vi "FTW-Test-Reflection-Datatypes.vi"() -> (0 "Test Result":errorcluster)   [LabVIEW 2014]
uses:
  src/core/reflection/FTW-Reflection-Types.ctl
  sandbox/deprecated/FTW-Collection-KeyValuePair.ctl
  src/core/actor/message/FTW-Message.lvclass
  src/core/database/FTW-SQLite-AccessMode.ctl
  src/core/error/FTW-ERR-ThrowError.vi
  src/core/error/FTW-ERR-Assert-DeveloperError.vi
  src/core/error/FTW-ERR-CallChain.vi
  src/core/string/FTW-STR-ReplaceWhitespace.vi
  src/core/database/FTW-SQLite-Connector.lvclass
panel:
  in  "DynamicData":dynamicdata(waveform)
  out "Results Array":T2(array[cluster])
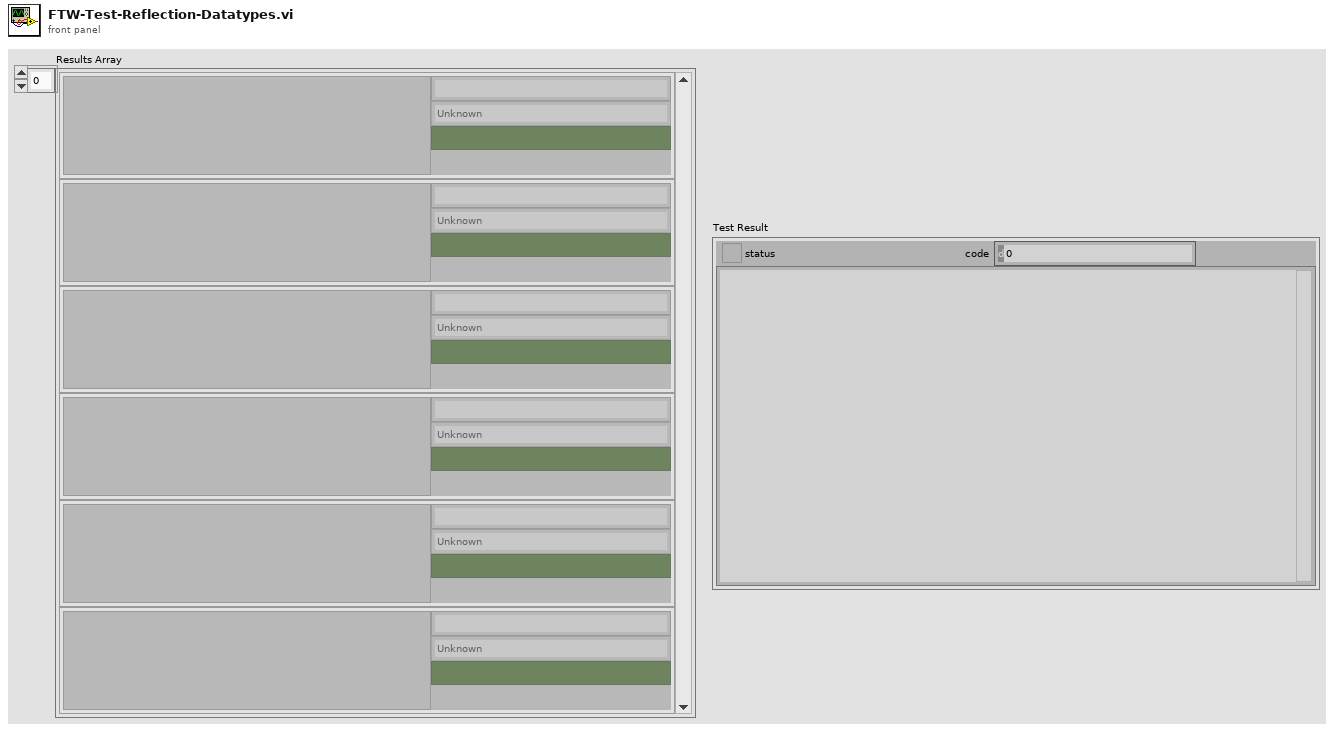
[diagram p1: front panel]
types:
  T1 = typedef "FTW-Reflection-Types.ctl" = enum16{"Unknown", "Void", "Array", "Cluster", "LVObject", "Boolean", "I8", "I16", "I32", "I64", "U8", "U16", "U32", "U64", "SGL", "DBL", "EXT", "CSG", "CDB", "CXT", "FXP", "EnumU8", "EnumU16", "EnumU32", "EnumU64", "SGLwithUnit", "DBLwithUnit", "EXTwithUnit", "CSGwithUnit", "CDBwithUnit", "CXTwithUnit", "String", "Path", "Picture", "Tag", "LVVariant", "Timestamp", "WaveformI8", "WaveformI16", "WaveformI32", "WaveformI64", "WaveformU8", "WaveformU16", "WaveformU32", "WaveformU64", "WaveformSGL", "WaveformDBL", "WaveformEXT", "WaveformCSG", "WaveformCDB", "WaveformCXT", "WaveformDigital", "WaveformUnknownType", "DigitalData", "DynamicData", "ExternalData", "FileByteStream", "TDMStream", "dotNET", "ActiveX", "VIServerReference", "VIReference", "ApplicationInstance", "Menu", "ConnectionDataSocket", "ConnectionVISA", "ConnectionBluetooth", "ConnectionIrDA", "ConnectionTCP", "ConnectionUDP", "ConnectionHTTPClient", "ConnectionFTP", "Occurrence", "Notifier", "Queue", "Rendezvous", "Semaphore", "RTFIFO", "EventPublisher", "EventRegistration", "EventCallback", "DataValueReference", "GenericClass", "GenericClassTag", "GenericClassDeepCopy", "GenericClassFlattened", "GenericClassTagFlattened", "GenericReferenceType", "WindowsRegistry", "OverloadedDatalogRef", "ReferenceUnknownType"}
  T2 = cluster{"Variant":variant, "xml string":string, "LabVIEW Type":T1, "Pass?":bool}[]
  T3 = typedef "Rendezvous RefNum" = refnum<k1>
  T4 = typedef "Semaphore RefNum" = refnum<k1>
  T5 = typedef "FTW-SQLite-Connector.lvclass/FTW-SQLite-AccessMode.ctl" = enum16{"Read", "Read/Write", "Read/Write/Create"}
  T6 = typedef "FTW-Collection-KeyValuePair.ctl" = cluster{"Key":string, "Value":string}
  T7 = cluster{"Variant":variant, "Match":string, "LabVIEW Type":T1, "Status OK?":bool}
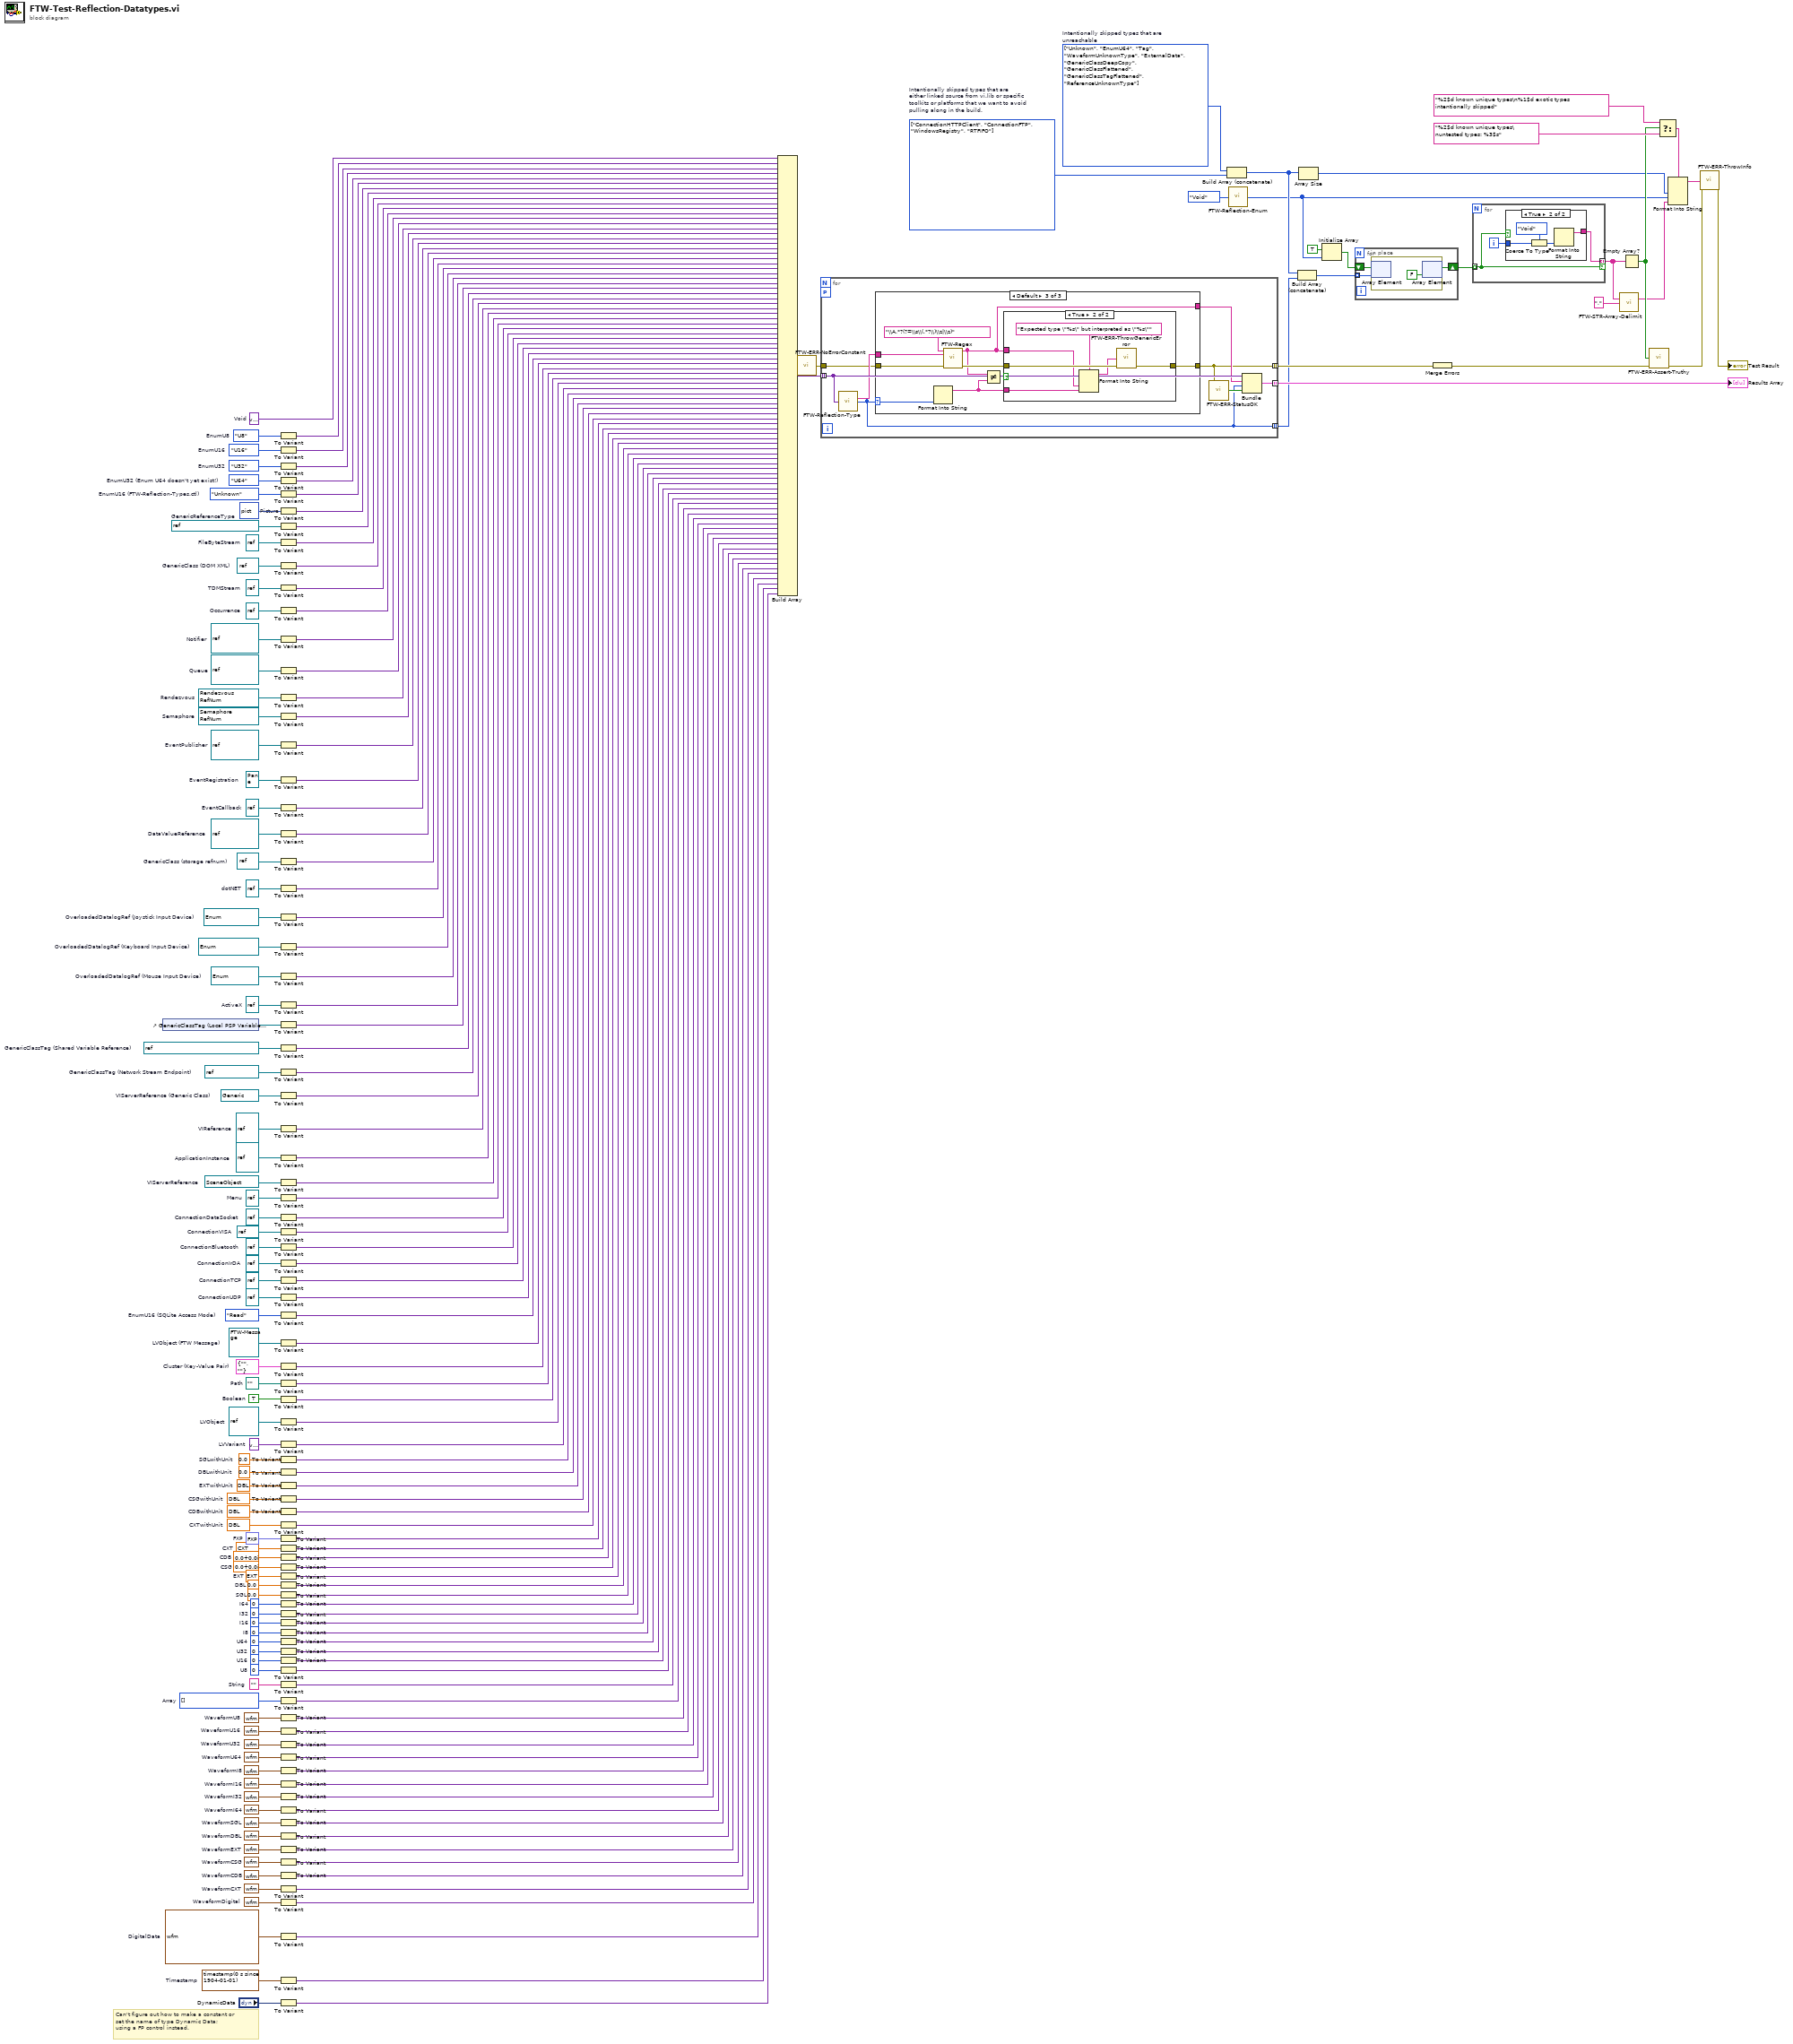
[diagram p0: block diagram]
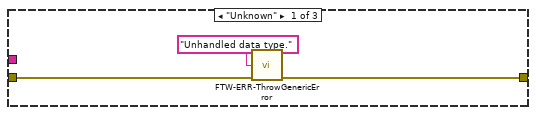
[diagram p3: hidden frame]
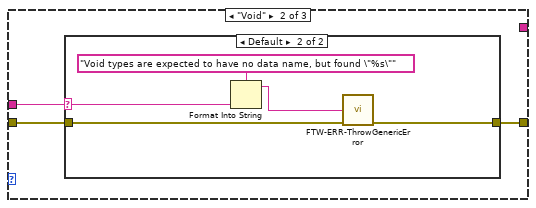
[diagram p4: hidden frame]
diagram:
  w19 = T1[] [enum."ConnectionHTTPClient", enum."ConnectionFTP", enum."WindowsRegistry", enum."RTFIFO"] items=["Unknown", "Void", "Array", "Cluster", "LVObject", "Boolean", "I8", "I16", "I32", "I64", "U8", "U16", "U32", "U64", "SGL", "DBL", "EXT", "CSG", "CDB", "CXT", "FXP", "EnumU8", "EnumU16", "EnumU32", "EnumU64", "SGLwithUnit", "DBLwithUnit", "EXTwithUnit", "CSGwithUnit", "CDBwithUnit", "CXTwithUnit", "String", "Path", "Picture", "Tag", "LVVariant", "Timestamp", "WaveformI8", "WaveformI16", "WaveformI32", "WaveformI64", "WaveformU8", "WaveformU16", "WaveformU32", "WaveformU64", "WaveformSGL", "WaveformDBL", "WaveformEXT", "WaveformCSG", "WaveformCDB", "WaveformCXT", "WaveformDigital", "WaveformUnknownType", "DigitalData", "DynamicData", "ExternalData", "FileByteStream", "TDMStream", "dotNET", "ActiveX", "VIServerReference", "VIReference", "ApplicationInstance", "Menu", "ConnectionDataSocket", "ConnectionVISA", "ConnectionBluetooth", "ConnectionIrDA", "ConnectionTCP", "ConnectionUDP", "ConnectionHTTPClient", "ConnectionFTP", "Occurrence", "Notifier", "Queue", "Rendezvous", "Semaphore", "RTFIFO", "EventPublisher", "EventRegistration", "EventCallback", "DataValueReference", "GenericClass", "GenericClassTag", "GenericClassDeepCopy", "GenericClassFlattened", "GenericClassTagFlattened", "GenericReferenceType", "WindowsRegistry", "OverloadedDatalogRef", "ReferenceUnknownType"]  # Intentionally skipped types that are either linked source from vi.lib or specific toolkits or platforms that we want to avoid pulling along in the build.
  w20 = T1[] [enum."Unknown", enum."EnumU64", enum."Tag", enum."WaveformUnknownType", enum."ExternalData", enum."GenericClassDeepCopy", enum."GenericClassFlattened", enum."GenericClassTagFlattened", enum."ReferenceUnknownType"] items=["Unknown", "Void", "Array", "Cluster", "LVObject", "Boolean", "I8", "I16", "I32", "I64", "U8", "U16", "U32", "U64", "SGL", "DBL", "EXT", "CSG", "CDB", "CXT", "FXP", "EnumU8", "EnumU16", "EnumU32", "EnumU64", "SGLwithUnit", "DBLwithUnit", "EXTwithUnit", "CSGwithUnit", "CDBwithUnit", "CXTwithUnit", "String", "Path", "Picture", "Tag", "LVVariant", "Timestamp", "WaveformI8", "WaveformI16", "WaveformI32", "WaveformI64", "WaveformU8", "WaveformU16", "WaveformU32", "WaveformU64", "WaveformSGL", "WaveformDBL", "WaveformEXT", "WaveformCSG", "WaveformCDB", "WaveformCXT", "WaveformDigital", "WaveformUnknownType", "DigitalData", "DynamicData", "ExternalData", "FileByteStream", "TDMStream", "dotNET", "ActiveX", "VIServerReference", "VIReference", "ApplicationInstance", "Menu", "ConnectionDataSocket", "ConnectionVISA", "ConnectionBluetooth", "ConnectionIrDA", "ConnectionTCP", "ConnectionUDP", "ConnectionHTTPClient", "ConnectionFTP", "Occurrence", "Notifier", "Queue", "Rendezvous", "Semaphore", "RTFIFO", "EventPublisher", "EventRegistration", "EventCallback", "DataValueReference", "GenericClass", "GenericClassTag", "GenericClassDeepCopy", "GenericClassFlattened", "GenericClassTagFlattened", "GenericReferenceType", "WindowsRegistry", "OverloadedDatalogRef", "ReferenceUnknownType"]  # Intentionally skipped types that are unreachable
  w24 = u8[] []  # Array
  w23 = ""  # String
  w12 = T3 refnum items=["rendezvous"]  # Rendezvous
  w11 = T4 refnum items=["semaphore"]  # Semaphore
  w27 = enum32{"U64"}."U64"  # EnumU32 (Enum U64 doesn't yet exist!)
  w37 = FTW-SQLite-AccessMode."Read"  # EnumU16 (SQLite Access Mode)
  w38 = refnum<class "FTW-Message.lvclass"> refnum  # LVObject (FTW Message)
  w41 = digitalwaveform {"t0"=timestamp(0 s since 1904-01-01), "dt"=0.0, "Y"={"transitions"=[], "data"=[]}}  # WaveformDigital
  w42 = waveform(cxt) {"t0"=timestamp(0 s since 1904-01-01), "dt"=1.0, "Y"=[]}  # WaveformCXT
  w43 = waveform(cdb) {"t0"=timestamp(0 s since 1904-01-01), "dt"=1.0, "Y"=[]}  # WaveformCDB
  w44 = waveform(csg) {"t0"=timestamp(0 s since 1904-01-01), "dt"=1.0, "Y"=[]}  # WaveformCSG
  w45 = waveform(ext) {"t0"=timestamp(0 s since 1904-01-01), "dt"=1.0, "Y"=[]}  # WaveformEXT
  w46 = waveform(dbl) {"t0"=timestamp(0 s since 1904-01-01), "dt"=1.0, "Y"=[]}  # WaveformDBL
  w47 = waveform(sgl) {"t0"=timestamp(0 s since 1904-01-01), "dt"=1.0, "Y"=[]}  # WaveformSGL
  w48 = waveform(i64) {"t0"=timestamp(0 s since 1904-01-01), "dt"=1.0, "Y"=[]}  # WaveformI64
  w49 = waveform(i32) {"t0"=timestamp(0 s since 1904-01-01), "dt"=1.0, "Y"=[]}  # WaveformI32
  w50 = waveform(i16) {"t0"=timestamp(0 s since 1904-01-01), "dt"=1.0, "Y"=[]}  # WaveformI16
  w54 = waveform(i8) {"t0"=timestamp(0 s since 1904-01-01), "dt"=1.0, "Y"=[]}  # WaveformI8
  w55 = waveform(u64) {"t0"=timestamp(0 s since 1904-01-01), "dt"=1.0, "Y"=[]}  # WaveformU64
  w53 = waveform(u32) {"t0"=timestamp(0 s since 1904-01-01), "dt"=1.0, "Y"=[]}  # WaveformU32
  w52 = waveform(u16) {"t0"=timestamp(0 s since 1904-01-01), "dt"=1.0, "Y"=[]}  # WaveformU16
  w51 = waveform(u8) {"t0"=timestamp(0 s since 1904-01-01), "dt"=1.0, "Y"=[]}  # WaveformU8
  w2 = variant  # Void
  w129 = refnum<k31> refnum  # ConnectionBluetooth
  w100 = enum32{"U32"}."U32"  # EnumU32
  w99 = enum16{"U16"}."U16"  # EnumU16
  w98 = enum8{"U8"}."U8"  # EnumU8
  w133 = TRUE  # Boolean
  w135 = path ""  # Path
  w101 = FTW-Reflection-Types."Unknown"  # EnumU16 (FTW-Reflection-Types.ctl)
  w109 = refnum<event-registration> refnum  # EventRegistration
  w134 = T6 {"Key"="", "Value"=""}  # Cluster (Key-Value Pair)
  w132 = refnum<k16> refnum  # ConnectionUDP
  w131 = refnum<k5> refnum  # ConnectionTCP
  w127 = refnum<k13> refnum  # ConnectionDataSocket
  w126 = refnum<k9> refnum  # Menu
  w111 = refnum<data-value> refnum  # DataValueReference
  w130 = refnum<k19> refnum  # ConnectionIrDA
  w102 = picture data[5B]  # Picture
  w125 = refnum<vi> refnum  # VIServerReference
  w123 = refnum<vi> refnum  # ApplicationInstance
  w124 = refnum<vi> refnum  # VIReference
  w122 = refnum<vi> refnum  # VIServerReference (Generic Class)
  w121 = refnum<k21> "localhost"  # GenericClassTag (Network Stream Endpoint)
  w112 = refnum<k27> refnum  # EventCallback
  w110 = refnum<user-event> refnum  # EventPublisher
  w107 = refnum<k4> refnum  # Occurrence
  w16 = refnum<queue> refnum  # Queue
  w108 = refnum<notifier> refnum  # Notifier
  w120 = refnum<k21> "ni.var.psp://localhost/System"  # GenericClassTag (Shared Variable Reference)
  w118 = refnum<k7> refnum  # ActiveX
  w117 = refnum<k1> refnum items=["MOUSE"]  # OverloadedDatalogRef (Mouse Input Device)
  w115 = refnum<k1> refnum items=["KEYBOARD"]  # OverloadedDatalogRef (Keyboard Input Device)
  w116 = refnum<k1> refnum items=["JOYSTICK"]  # OverloadedDatalogRef (Joystick Input Device)
  w113 = refnum<k24> refnum  # dotNET
  w114 = refnum<k20> refnum  # GenericClass (storage refnum)
  w106 = refnum<k34> refnum  # TDMStream
  w103 = refnum<k0> refnum  # GenericReferenceType
  w128 = refnum<visa-resource-name> refnum  # ConnectionVISA
  w105 = refnum<k20> refnum  # GenericClass (DOM XML)
  w104 = refnum<file> refnum  # FileByteStream
  w137 = refnum<class> refnum  # LVObject
  w139 = variant  # LVVariant
  w151 = cxt[unit] 0.0+0.0i  # CXTwithUnit
  w150 = cdb[unit] 0.0+0.0i  # CDBwithUnit
  w149 = csg[unit] 0.0+0.0i  # CSGwithUnit
  w148 = ext[unit] 0.0  # EXTwithUnit
  w147 = dbl[unit] 0.0  # DBLwithUnit
  w146 = sgl[unit] 0.0  # SGLwithUnit
  w198 = timestamp(0 s since 1904-01-01)  # Timestamp
  w168 = cxt 0.0+0.0i  # CXT
  w169 = cdb 0.0+0.0i  # CDB
  w170 = csg 0.0+0.0i  # CSG
  w167 = fxp<+/-,64,1024> 0.0  # FXP
  w171 = ext 0.0  # EXT
  w172 = 0.0  # DBL
  w173 = sgl 0.0  # SGL
  w174 = i64 0  # I64
  w175 = 0  # I32
  w176 = i16 0  # I16
  w177 = i8 0  # I8
  w178 = u64 0  # U64
  w179 = u32 0  # U32
  w180 = u16 0  # U16
  w181 = u8 0  # U8
  w201 = digitaldata {"transitions"=[], "data"=[]}  # DigitalData
  # "Can't figure out how to make a constant or\nset the name of type Dynamic Data;\nusing a FP control instead."
  n1 = control-ref of="GenericClassTag (Local PSP Variable Engine)"() -> (w119:refnum<k21>)
  n2 = To Variant(anything=w98) -> (Variant=w1:variant)
  n3 = To Variant(anything=w99) -> (Variant=w57:variant)
  n4 = To Variant(anything=w100) -> (Variant=w25:variant)
  n5 = To Variant(anything=w27) -> (Variant=w26:variant)
  n6 = To Variant(anything=w101) -> (Variant=w58:variant)
  n7 = To Variant(anything=w102) -> (Variant=w59:variant)
  n8 = To Variant(anything=w103) -> (Variant=w60:variant)
  n9 = To Variant(anything=w104) -> (Variant=w61:variant)
  n10 = To Variant(anything=w105) -> (Variant=w62:variant)
  n11 = To Variant(anything=w106) -> (Variant=w63:variant)
  n12 = To Variant(anything=w107) -> (Variant=w64:variant)
  n13 = To Variant(anything=w108) -> (Variant=w65:variant)
  n14 = To Variant(anything=w16) -> (Variant=w66:variant)
  n15 = To Variant(anything=w12) -> (Variant=w67:variant)
  n16 = To Variant(anything=w11) -> (Variant=w68:variant)
  n17 = To Variant(anything=w110) -> (Variant=w69:variant)
  n18 = To Variant(anything=w109) -> (Variant=w70:variant)
  n19 = To Variant(anything=w112) -> (Variant=w71:variant)
  n20 = To Variant(anything=w111) -> (Variant=w72:variant)
  n21 = To Variant(anything=w114) -> (Variant=w73:variant)
  n22 = To Variant(anything=w113) -> (Variant=w74:variant)
  n23 = To Variant(anything=w116) -> (Variant=w75:variant)
  n24 = To Variant(anything=w115) -> (Variant=w76:variant)
  n25 = To Variant(anything=w117) -> (Variant=w77:variant)
  n26 = To Variant(anything=w118) -> (Variant=w78:variant)
  n27 = To Variant(anything=w119) -> (Variant=w79:variant)
  n28 = To Variant(anything=w120) -> (Variant=w80:variant)
  n29 = To Variant(anything=w121) -> (Variant=w81:variant)
  n30 = To Variant(anything=w122) -> (Variant=w82:variant)
  n31 = To Variant(anything=w124) -> (Variant=w83:variant)
  n32 = To Variant(anything=w123) -> (Variant=w84:variant)
  n33 = To Variant(anything=w125) -> (Variant=w85:variant)
  n34 = To Variant(anything=w126) -> (Variant=w86:variant)
  n35 = To Variant(anything=w127) -> (Variant=w87:variant)
  n36 = To Variant(anything=w128) -> (Variant=w88:variant)
  n37 = To Variant(anything=w129) -> (Variant=w89:variant)
  n38 = To Variant(anything=w130) -> (Variant=w90:variant)
  n39 = To Variant(anything=w131) -> (Variant=w91:variant)
  n40 = To Variant(anything=w132) -> (Variant=w92:variant)
  n41 = To Variant(anything=w37) -> (Variant=w93:variant)
  n42 = To Variant(anything=w38) -> (Variant=w94:variant)
  n43 = To Variant(anything=w134) -> (Variant=w95:variant)
  n44 = To Variant(anything=w135) -> (Variant=w96:variant)
  n45 = To Variant(anything=w133) -> (Variant=w97:variant)
  n46 = To Variant(anything=w137) -> (Variant=w136:variant)
  n47 = To Variant(anything=w139) -> (Variant=w138:variant)
  n48 = To Variant(anything=w146) -> (Variant=w140:variant)
  n49 = To Variant(anything=w147) -> (Variant=w141:variant)
  n50 = To Variant(anything=w148) -> (Variant=w142:variant)
  n51 = To Variant(anything=w149) -> (Variant=w143:variant)
  n52 = To Variant(anything=w150) -> (Variant=w144:variant)
  n53 = To Variant(anything=w151) -> (Variant=w145:variant)
  n54 = To Variant(anything=w167) -> (Variant=w152:variant)
  n55 = To Variant(anything=w168) -> (Variant=w153:variant)
  n56 = To Variant(anything=w169) -> (Variant=w154:variant)
  n57 = To Variant(anything=w170) -> (Variant=w155:variant)
  n58 = To Variant(anything=w171) -> (Variant=w156:variant)
  n59 = To Variant(anything=w172) -> (Variant=w157:variant)
  n60 = To Variant(anything=w173) -> (Variant=w158:variant)
  n61 = To Variant(anything=w174) -> (Variant=w159:variant)
  n62 = To Variant(anything=w175) -> (Variant=w160:variant)
  n63 = To Variant(anything=w176) -> (Variant=w161:variant)
  n64 = To Variant(anything=w177) -> (Variant=w162:variant)
  n65 = To Variant(anything=w178) -> (Variant=w163:variant)
  n66 = To Variant(anything=w179) -> (Variant=w164:variant)
  n67 = To Variant(anything=w180) -> (Variant=w165:variant)
  n68 = To Variant(anything=w181) -> (Variant=w166:variant)
  n69 = To Variant(anything=w23) -> (Variant=w22:variant)
  n70 = To Variant(anything=w24) -> (Variant=w21:variant)
  n71 = To Variant(anything=w51) -> (Variant=w197:variant)
  n72 = To Variant(anything=w52) -> (Variant=w196:variant)
  n73 = To Variant(anything=w53) -> (Variant=w195:variant)
  n74 = To Variant(anything=w55) -> (Variant=w194:variant)
  n75 = To Variant(anything=w54) -> (Variant=w193:variant)
  n76 = To Variant(anything=w50) -> (Variant=w192:variant)
  n77 = To Variant(anything=w49) -> (Variant=w191:variant)
  n78 = To Variant(anything=w48) -> (Variant=w190:variant)
  n79 = To Variant(anything=w47) -> (Variant=w189:variant)
  n80 = To Variant(anything=w46) -> (Variant=w188:variant)
  n81 = To Variant(anything=w45) -> (Variant=w187:variant)
  n82 = To Variant(anything=w44) -> (Variant=w186:variant)
  n83 = To Variant(anything=w43) -> (Variant=w185:variant)
  n84 = To Variant(anything=w42) -> (Variant=w184:variant)
  n85 = To Variant(anything=w41) -> (Variant=w183:variant)
  n86 = To Variant(anything=w201) -> (Variant=w182:variant)
  n87 = To Variant(anything=w198) -> (Variant=w56:variant)
  n88 = To Variant(anything="DynamicData") -> (Variant=w40:variant)
  n89 = Build Array(w2, w1, w57, w25, w26, w58, w59, w60, w61, w62, w63, w64, w65, w66, w67, w68, w69, w70, w71, w72, w73, w74, w75, w76, w77, w78, w79, w80, w81, w82, w83, w84, w85, w86, w87, w88, w89, w90, w91, w92, w93, w94, w95, w96, w97, w136, w138, w140, w141, w142, w143, w144, w145, w152, w153, w154, w155, w156, w157, w158, w159, w160, w161, w162, w163, w164, w165, w166, w22, w21, w197, w196, w195, w194, w193, w192, w191, w190, w189, w188, w187, w186, w185, w184, w183, w182, w56, w40) -> (w199:variant[])
  n90 = call "FTW-ERR-NoErrorConstant.vi"() -> ("no error"=w36:errorcluster)
  n91 = for {
    tunnel: w199 -> [w208] mode=indexing
    tunnel: [w209] -> w200 mode=indexing
    tunnel: w36 -> [w206]
    workers-P: _ -> [_]
    tunnel: [w204] -> w35 mode=indexing
    tunnel: [w202] -> w10 mode=indexing
    n92 = call "FTW-Reflection-Type.vi"("Anything"=w208) -> ("Data Name"=w207:string, "LabVIEW Type"=w202:T1)  [unwired: 12 in, 1 out]
    n93 = case shown="Default" w202 {
      selector: w202 -> [_ _ w227]
      tunnel: w207 -> [_ w213 w230]
      tunnel: w206 -> [w211 w215 w229]
      tunnel: [w210 w214 w224] -> w204
      tunnel: [_ _ w222] -> w205
      frame "Unknown" {
        n94 = call "FTW-ERR-ThrowGenericError.vi"("Error Message"="Unhandled data type.", "error in"=w211) -> ("error out"=w210:errorcluster)  [unwired: 13 in]
      }
      frame "Void" {
        n95 = case shown="Default" w213 {
          selector: w213 -> [_ w217]
          tunnel: w215 -> [w216 w221]
          tunnel: [w216 w220] -> w214
          frame "" {
          }
          frame Default {
            n96 = Format Into String(format string="Void types are expected to have no data name, but found \"%s\"", w217) -> (resulting string=w218:string)  [unwired: 2 in, 1 out]
            n97 = call "FTW-ERR-ThrowGenericError.vi"("Error Message"=w218, "error in"=w221) -> ("error out"=w220:errorcluster)  [unwired: 13 in]
          }
        }
      }
      frame Default {
        n98 = Format Into String(w227) -> (resulting string=w223:string)  [unwired: 3 in, 1 out]
        n99 = call "FTW-Regex.vi"("Regular Expression"="\\A.*?(?=\\s\\(.*?\\)\\z|\\z)", "Input String"=w230, "error in"=w229) -> ("Match"=w222:string, "error out"=w225:errorcluster)  [unwired: 8 in, 3 out]
        n100 = Not Equal?(x=w222, y=w223) -> (x != y?=w226:bool)
        n101 = case shown="True" w226 {
          tunnel: w225 -> [w231 w237]
          tunnel: [w231 w236] -> w224
          tunnel: w222 -> [_ w235]
          tunnel: w223 -> [_ w234]
          frame False {
          }
          frame True {
            n102 = Format Into String(format string="Expected type \"%s\" but interpreted as \"%s\"", w235, w234) -> (resulting string=w232:string)  [unwired: 2 in, 1 out]
            n103 = call "FTW-ERR-ThrowGenericError.vi"("Error Message"=w232, "error in"=w237) -> ("error out"=w236:errorcluster)  [unwired: 13 in]
          }
        }
      }
    }
    n104 = call "FTW-ERR-StatusOK.vi"("error to check"=w204) -> ("Status OK?"=w203:bool)
    n105 = Bundle("Variant"=w208, "Match"=w205, "LabVIEW Type"=w202, "Status OK?"=w203) -> (w209:T7)  [unwired: 1 in]
  }
  "Results Array" <- w200
  n106 = Build Array (concatenate)(w20, w19) -> (w17:T1[])
  n107 = call "FTW-Reflection-Enum.vi"("Enum"=FTW-Reflection-Types."Void" ("y")) -> ("Number of Items"=w4:i32)  [unwired: 12 in, 2 out]
  n108 = Build Array (concatenate)(w17, w10) -> (w18:T1[])
  n109 = Array Size(array=w17) -> (size(s)=w3:i32)
  n110 = Initialize Array(TRUE, w4) -> (w29:bool[])
  n111 = for {
    shift-right: [w239] -> w28
    shift-left: w29 -> [w240]
    tunnel: w18 -> [w238] mode=indexing
    n112 = in-place {
      n113 = in-place-array #1(w240, w238) -> ()  [unwired: 1 out]
      n114 = in-place-array #1(FALSE ("element")) -> (w239:bool[])  [unwired: 1 out]
    }
  }
  n115 = Merge Errors(w35) -> (w15:errorcluster)
  n116 = for {
    tunnel: w28 -> [w242] mode=indexing
    tunnel: [w243] -> w31 mode=indexing if=w242
    i -> [w244]
    n117 = case shown="True" w242 {
      tunnel: w244 -> [_ w248]
      tunnel: [_ w246] -> w243
      frame False {
      }
      frame True {
        n118 = Coerce To Type(0:w248, 1:FTW-Reflection-Types."Void" ("y")) -> (2:w247:T1)
        n119 = Format Into String(w247) -> (resulting string=w246:string)  [unwired: 3 in, 1 out]
      }
    }
  }
  n120 = call "FTW-STR-Array-Delimit.vi"("Array of Strings"=w31, "Delimiter"=",") -> ("Delimited String"=w5:string)  [unwired: 13 in]
  n121 = Empty Array?(array=w31) -> (empty?=w8:bool)
  n122 = call "FTW-ERR-Assert-Truthy.vi"("Expected Truthy"=w8, "error in"=w15) -> ("error out"=w14:errorcluster)  [unwired: 13 in]
  n123 = Select(t="%2$d known unique types\n%1$d exotic types intentionally skipped" ("format string"), s=w8, f="%2$d known unique types\nuntested types: %3$s" ("format string")) -> (s? t:f=w6:string)
  n124 = Format Into String(format string=w6, w3, w4, w5) -> (resulting string=w32:string)  [unwired: 2 in, 1 out]
  n125 = call "FTW-ERR-ThrowInfo.vi"("Informational Message"=w32, "error in"=w14) -> ("error out"=→"Test Result":errorcluster)  [unwired: 13 in]
